vi "校准参数读取.vi"(8 "error in":errorcluster caption="错误输入", 11 "Channel":u16=81 format="%.0x") -> (0 "error out":errorcluster caption="错误输出", 1 "斜率":i32, 2 "截距":i32)   [LabVIEW 2020]
uses:
  <userlib>/PCANBasic/ctl/TPCANStatus.ctl
  <userlib>/PCANBasic/ctl/TPCANMsgFD.ctl
  <userlib>/PCANBasic/PCANBasic.lvlib
panel:
  out "TCANStatus 4":T1 items=["PCAN_ERROR_OK"=0, "PCAN_ERROR_XMTFULL"=1, "PCAN_ERROR_OVERRUN"=2, "PCAN_ERROR_BUSLIGHT"=4, "PCAN_ERROR_BUSHEAVY"=8, "PCAN_ERROR_BUSPASSIVE"=262144, "PCAN_ERROR_BUSOFF"=16, "PCAN_ERROR_QRCVEMPTY"=32, "PCAN_ERROR_QOVERRUN"=64, "PCAN_ERROR_QXMTFULL"=128, "PCAN_ERROR_REGTEST"=256, "PCAN_ERROR_NODRIVER"=512, "PCAN_ERROR_HWINUSE"=1024, "PCAN_ERROR_NETINUSE"=2048, "PCAN_ERROR_ILLHW"=5120, "PCAN_ERROR_ILLNET"=6144, "PCAN_ERROR_ILLCLIENT"=7168, "PCAN_ERROR_RESOURCE"=8192, "PCAN_ERROR_ILLPARAMTYPE"=16384, "PCAN_ERROR_ILLPARAMVAL"=32768, "PCAN_ERROR_UNKNOWN"=65536, "PCAN_ERROR_ILLDATA"=131072, "PCAN_ERROR_CAUTION"=33554432, "PCAN_ERROR_INITIALIZE"=67108864, "PCAN_ERROR_ILLOPERATION"=134217728]
  out "TCANStatus 3":T1 items=["PCAN_ERROR_OK"=0, "PCAN_ERROR_XMTFULL"=1, "PCAN_ERROR_OVERRUN"=2, "PCAN_ERROR_BUSLIGHT"=4, "PCAN_ERROR_BUSHEAVY"=8, "PCAN_ERROR_BUSPASSIVE"=262144, "PCAN_ERROR_BUSOFF"=16, "PCAN_ERROR_QRCVEMPTY"=32, "PCAN_ERROR_QOVERRUN"=64, "PCAN_ERROR_QXMTFULL"=128, "PCAN_ERROR_REGTEST"=256, "PCAN_ERROR_NODRIVER"=512, "PCAN_ERROR_HWINUSE"=1024, "PCAN_ERROR_NETINUSE"=2048, "PCAN_ERROR_ILLHW"=5120, "PCAN_ERROR_ILLNET"=6144, "PCAN_ERROR_ILLCLIENT"=7168, "PCAN_ERROR_RESOURCE"=8192, "PCAN_ERROR_ILLPARAMTYPE"=16384, "PCAN_ERROR_ILLPARAMVAL"=32768, "PCAN_ERROR_UNKNOWN"=65536, "PCAN_ERROR_ILLDATA"=131072, "PCAN_ERROR_CAUTION"=33554432, "PCAN_ERROR_INITIALIZE"=67108864, "PCAN_ERROR_ILLOPERATION"=134217728]
  out "TCANStatus 2":T1 items=["PCAN_ERROR_OK"=0, "PCAN_ERROR_XMTFULL"=1, "PCAN_ERROR_OVERRUN"=2, "PCAN_ERROR_BUSLIGHT"=4, "PCAN_ERROR_BUSHEAVY"=8, "PCAN_ERROR_BUSPASSIVE"=262144, "PCAN_ERROR_BUSOFF"=16, "PCAN_ERROR_QRCVEMPTY"=32, "PCAN_ERROR_QOVERRUN"=64, "PCAN_ERROR_QXMTFULL"=128, "PCAN_ERROR_REGTEST"=256, "PCAN_ERROR_NODRIVER"=512, "PCAN_ERROR_HWINUSE"=1024, "PCAN_ERROR_NETINUSE"=2048, "PCAN_ERROR_ILLHW"=5120, "PCAN_ERROR_ILLNET"=6144, "PCAN_ERROR_ILLCLIENT"=7168, "PCAN_ERROR_RESOURCE"=8192, "PCAN_ERROR_ILLPARAMTYPE"=16384, "PCAN_ERROR_ILLPARAMVAL"=32768, "PCAN_ERROR_UNKNOWN"=65536, "PCAN_ERROR_ILLDATA"=131072, "PCAN_ERROR_CAUTION"=33554432, "PCAN_ERROR_INITIALIZE"=67108864, "PCAN_ERROR_ILLOPERATION"=134217728]
  out "TCANStatus":T1 items=["PCAN_ERROR_OK"=0, "PCAN_ERROR_XMTFULL"=1, "PCAN_ERROR_OVERRUN"=2, "PCAN_ERROR_BUSLIGHT"=4, "PCAN_ERROR_BUSHEAVY"=8, "PCAN_ERROR_BUSPASSIVE"=262144, "PCAN_ERROR_BUSOFF"=16, "PCAN_ERROR_QRCVEMPTY"=32, "PCAN_ERROR_QOVERRUN"=64, "PCAN_ERROR_QXMTFULL"=128, "PCAN_ERROR_REGTEST"=256, "PCAN_ERROR_NODRIVER"=512, "PCAN_ERROR_HWINUSE"=1024, "PCAN_ERROR_NETINUSE"=2048, "PCAN_ERROR_ILLHW"=5120, "PCAN_ERROR_ILLNET"=6144, "PCAN_ERROR_ILLCLIENT"=7168, "PCAN_ERROR_RESOURCE"=8192, "PCAN_ERROR_ILLPARAMTYPE"=16384, "PCAN_ERROR_ILLPARAMVAL"=32768, "PCAN_ERROR_UNKNOWN"=65536, "PCAN_ERROR_ILLDATA"=131072, "PCAN_ERROR_CAUTION"=33554432, "PCAN_ERROR_INITIALIZE"=67108864, "PCAN_ERROR_ILLOPERATION"=134217728]
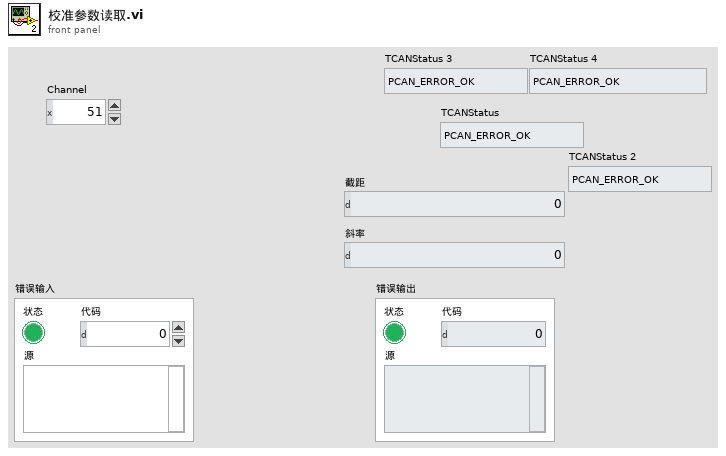
[diagram p1: front panel]
types:
  T1 = typedef "PCANBasic.lvlib/TPCANStatus.ctl" = u32
  T2 = typedef "PCANBasic.lvlib/TPCANMsgFD.ctl" = cluster{"ID":u32, "MSGTYPE":u8, "DLC":u8, "DATA":cluster{"[0]":u8, "[1]":u8, "[2]":u8, "[3]":u8, "[4]":u8, "[5]":u8, "[6]":u8, "[7]":u8, "[8]":u8, "[9]":u8, "[10]":u8, "[11]":u8, "[12]":u8, "[13]":u8, "[14]":u8, "[15]":u8, "[16]":u8, "[17]":u8, "[18]":u8, "[19]":u8, "[20]":u8, "[21]":u8, "[22]":u8, "[23]":u8, "[24]":u8, "[25]":u8, "[26]":u8, "[27]":u8, "[28]":u8, "[29]":u8, "[30]":u8, "[31]":u8, "[32]":u8, "[33]":u8, "[34]":u8, "[35]":u8, "[36]":u8, "[37]":u8, "[38]":u8, "[39]":u8, "[40]":u8, "[41]":u8, "[42]":u8, "[43]":u8, "[44]":u8, "[45]":u8, "[46]":u8, "[47]":u8, "[48]":u8, "[49]":u8, "[50]":u8, "[51]":u8, "[52]":u8, "[53]":u8, "[54]":u8, "[55]":u8, "[56]":u8, "[57]":u8, "[58]":u8, "[59]":u8, "[60]":u8, "[61]":u8, "[62]":u8, "[63]":u8}}
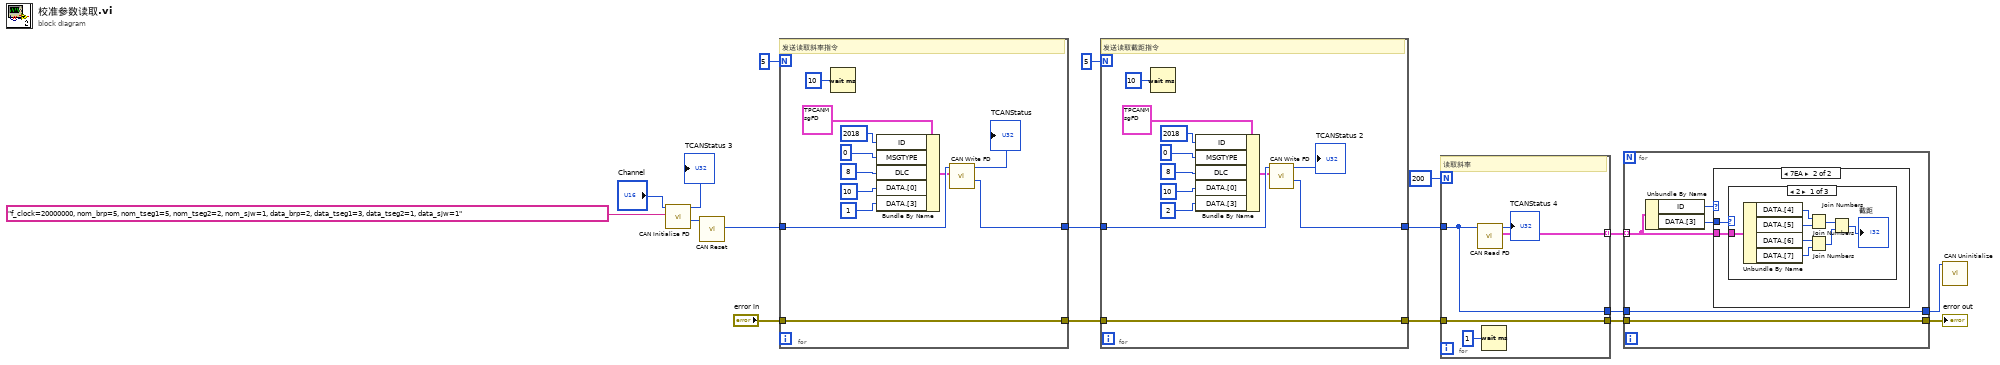
[diagram p0: block diagram]
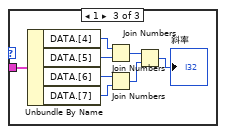
[diagram p4: hidden frame]
diagram:
  n1 = call <userlib>:"CAN Initialize FD.vi"("BitrateFD"="f_clock=20000000, nom_brp=5, nom_tseg1=5, nom_tseg2=2, nom_sjw=1, data_brp=2, data_tseg1=3, data_tseg2=1, data_sjw=1", "Channel"="Channel") -> ("Channel out"=w12:u16, "TCANStatus"=→"TCANStatus 3":T1)  [unwired: 6 in, 2 out]
  n2 = call <userlib>:"CAN Reset.vi"("Channel in"=w12) -> ("Channel out"=w11:u16)  [unwired: 8 in, 2 out]
  n3 = for {
    N: 5 -> [_]
    tunnel: w11 -> [w27]
    tunnel: [w19] -> w10
    tunnel: "error in" -> [w21]
    tunnel: [w21] -> w6
    # "发送读取斜率指令"
    n4 = Wait (ms)(milliseconds to wait=u32 10 ("等待时间（毫秒）")) -> ()  [unwired: 1 out]
    n5 = Bundle By Name(cluster=T2 {"ID"=0, "MSGTYPE"=0, "DLC"=0, "DATA"={"[0]"=0, "[1]"=0, "[2]"=0, "[3]"=0, "[4]"=0, "[5]"=0, "[6]"=0, "[7]"=0, "[8]"=0, "[9]"=0, "[10]"=0, "[11]"=0, "[12]"=0, "[13]"=0, "[14]"=0, "[15]"=0, "[16]"=0, "[17]"=0, "[18]"=0, "[19]"=0, "[20]"=0, "[21]"=0, "[22]"=0, "[23]"=0, "[24]"=0, "[25]"=0, "[26]"=0, "[27]"=0, "[28]"=0, "[29]"=0, "[30]"=0, "[31]"=0, "[32]"=0, "[33]"=0, "[34]"=0, "[35]"=0, "[36]"=0, "[37]"=0, "[38]"=0, "[39]"=0, "[40]"=0, "[41]"=0, "[42]"=0, "[43]"=0, "[44]"=0, "[45]"=0, "[46]"=0, "[47]"=0, "[48]"=0, "[49]"=0, "[50]"=0, "[51]"=0, "[52]"=0, "[53]"=0, "[54]"=0, "[55]"=0, "[56]"=0, "[57]"=0, "[58]"=0, "[59]"=0, "[60]"=0, "[61]"=0, "[62]"=0, "[63]"=0}} ("MessageBuffer"), "ID"=u32 2018, "MSGTYPE"=u8 0, "DLC"=u8 8 ("ID"), "DATA.[0]"=u8 10 ("ID"), "DATA.[3]"=u8 1 ("DATA[3]")) -> (w22:T2)
    n6 = call <userlib>:"CAN Write FD.vi"("MessageBuffer in"=w22, "Channel"=w27) -> ("Channel out"=w19:u16, "TCANStatus"=→"TCANStatus":T1)  [unwired: 6 in, 2 out]
  }
  n7 = for {
    N: 5 -> [_]
    tunnel: w10 -> [w39]
    tunnel: [w31] -> w9
    tunnel: w6 -> [w33]
    tunnel: [w33] -> w5
    # "发送读取截距指令"
    n8 = Wait (ms)(milliseconds to wait=u32 10 ("等待时间（毫秒）")) -> ()  [unwired: 1 out]
    n9 = Bundle By Name(cluster=T2 {"ID"=0, "MSGTYPE"=0, "DLC"=0, "DATA"={"[0]"=0, "[1]"=0, "[2]"=0, "[3]"=0, "[4]"=0, "[5]"=0, "[6]"=0, "[7]"=0, "[8]"=0, "[9]"=0, "[10]"=0, "[11]"=0, "[12]"=0, "[13]"=0, "[14]"=0, "[15]"=0, "[16]"=0, "[17]"=0, "[18]"=0, "[19]"=0, "[20]"=0, "[21]"=0, "[22]"=0, "[23]"=0, "[24]"=0, "[25]"=0, "[26]"=0, "[27]"=0, "[28]"=0, "[29]"=0, "[30]"=0, "[31]"=0, "[32]"=0, "[33]"=0, "[34]"=0, "[35]"=0, "[36]"=0, "[37]"=0, "[38]"=0, "[39]"=0, "[40]"=0, "[41]"=0, "[42]"=0, "[43]"=0, "[44]"=0, "[45]"=0, "[46]"=0, "[47]"=0, "[48]"=0, "[49]"=0, "[50]"=0, "[51]"=0, "[52]"=0, "[53]"=0, "[54]"=0, "[55]"=0, "[56]"=0, "[57]"=0, "[58]"=0, "[59]"=0, "[60]"=0, "[61]"=0, "[62]"=0, "[63]"=0}} ("MessageBuffer"), "ID"=u32 2018, "MSGTYPE"=u8 0, "DLC"=u8 8 ("ID"), "DATA.[0]"=u8 10 ("ID"), "DATA.[3]"=u8 2 ("DATA[3]")) -> (w34:T2)
    n10 = call <userlib>:"CAN Write FD.vi"("MessageBuffer in"=w34, "Channel"=w39) -> ("Channel out"=w31:u16, "TCANStatus"=→"TCANStatus 2":T1)  [unwired: 6 in, 2 out]
  }
  n11 = for {
    N: 200 -> [_]
    tunnel: w9 -> [w46]
    tunnel: [w46] -> w16
    tunnel: w5 -> [w45]
    tunnel: [w45] -> w4
    tunnel: [w44] -> w2 mode=indexing
    # "读取斜率"
    n12 = call <userlib>:"CAN Read FD.vi"("Channel"=w46) -> ("MessageBuffer out"=w44:T2, "TCANStatus"=→"TCANStatus 4":T1)  [unwired: 7 in, 2 out]
    n13 = Wait (ms)(milliseconds to wait=u32 1 ("等待时间（毫秒）")) -> ()  [unwired: 1 out]
  }
  n14 = for {
    tunnel: [w52] -> w15
    tunnel: w16 -> [w52]
    tunnel: w4 -> [w51]
    tunnel: [w51] -> w3
    tunnel: w2 -> [w48] mode=indexing
    n15 = Unbundle By Name(w48) -> ("ID"=w50:u32, "DATA.[3]"=w49:u8)
    n16 = case shown="7EA" w50 {
      tunnel: w48 -> [_ w54]
      tunnel: w49 -> [_ w53]
      frame 0, Default {
      }
      frame 2026 {
        n17 = case shown="2" w53 {
          tunnel: w54 -> [w55 _ w70]
          frame 2 {
            n18 = Unbundle By Name(w55) -> ("DATA.[4]"=w62:u8, "DATA.[5]"=w61:u8, "DATA.[6]"=w60:u8, "DATA.[7]"=w59:u8)
            n19 = Join Numbers(hi=w62, lo=w61) -> ((hi.lo)=w57:u16)
            n20 = Join Numbers(hi=w60, lo=w59) -> ((hi.lo)=w58:u16)
            n21 = Join Numbers(hi=w57, lo=w58) -> ((hi.lo)=→"截距":u32)
          }
          frame 3, Default {
          }
          frame 1 {
            n22 = Unbundle By Name(w70) -> ("DATA.[4]"=w69:u8, "DATA.[5]"=w68:u8, "DATA.[6]"=w67:u8, "DATA.[7]"=w66:u8)
            n23 = Join Numbers(hi=w69, lo=w68) -> ((hi.lo)=w64:u16)
            n24 = Join Numbers(hi=w67, lo=w66) -> ((hi.lo)=w65:u16)
            n25 = Join Numbers(hi=w64, lo=w65) -> ((hi.lo)=→"斜率":u32)
          }
        }
      }
    }
  }
  "error out" <- w3
  n26 = call <userlib>:"CAN Uninitialize.vi"("Channel"=w15) -> ()  [unwired: 10 in, 1 out]
